vi "ShowData.vi"(11 "PipeData in":refnum<class "StreamData.lvclass">) -> (0 "pipe data":cluster{"element":T1}[](array[cluster]), 1 "size":i32, 2 "count":i32, 3 "PipeData out":refnum<class "StreamData.lvclass">, 4 "last element":bool, 5 "abort":bool, 6 "unbounded":bool, 7 "OpCount":u32)   [LabVIEW 2017, in "Stream-t'WPI_EncoderType.ctl'.lvlib" / "StreamData.lvclass"]
uses:
  <extravilib>/ChannelInstances/Stream-t'WPI_EncoderType.ctl'/StreamData.lvclass
  <vilib>/Rock Robotics/WPI/Encoder/WPI_EncoderType.ctl
  <extravilib>/ChannelInstances/Stream-t'WPI_EncoderType.ctl'/StreamData.lvclass/StreamData.ctl
  <resource>/ChannelSupport/_ChannelSupport/PipeLogic/PipeLogic.lvclass/PipeLogic.ctl
  <resource>/ChannelSupport/_ChannelSupport/PipeLogic/PipeLogic.lvclass
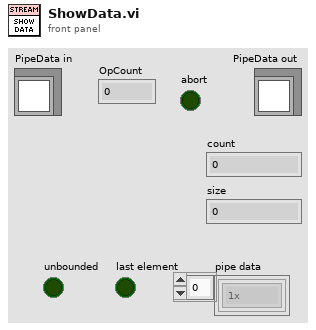
[diagram p1: front panel]
types:
  T1 = typedef "WPI_EncoderType.ctl" = enum16{"1x", "2x", "4x"}
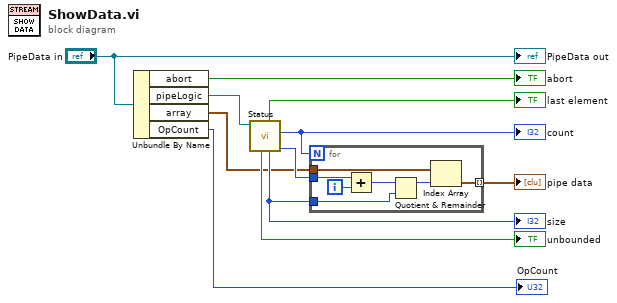
[diagram p0: block diagram]
diagram:
  n1 = Unbundle By Name("PipeData in") -> ("abort"=→"abort":bool, "pipeLogic"=w3:refnum<class "PipeLogic.lvclass">, "array"=w2:cluster{"element":T1}[], "OpCount"=→"OpCount":u32)
  n2 = call <resource>:"Status.vi"("pipeLogic in"=w3) -> ("index out"=w10:i32, "count"=w8:i32, "size"=w6:i32, "last element"=→"last element":bool, "unbounded"=→"unbounded":bool)  [unwired: 2 in, 4 out]
  "count" <- w8
  "size" <- w6
  n3 = for {
    N: w8 -> [_]
    tunnel: w2 -> [w18]
    tunnel: w10 -> [w17]
    tunnel: [w13] -> w7 mode=indexing
    tunnel: w6 -> [w12]
    i -> [w16]
    n4 = Add(x=w17, y=w16) -> (x+y=w15:i32)
    n5 = Quotient & Remainder(x=w15, y=w12) -> (x-y*floor(x/y)=w14:i32)  [unwired: 1 out]
    n6 = Index Array(array=w18, index=w14) -> (element=w13:cluster{"element":T1})
  }
  "pipe data" <- w7
  "PipeData out" <- "PipeData in"
